vi "LabVIEW.vi"() -> ()   [LabVIEW 2022 SP3]
uses:
  <vilib>/Analysis/NI_AALBase.lvlib
  <vilib>/Analysis/baseanly.llb/Mean (DBL).vi
  Humidity_Global.vi
  <vilib>/Instr/_visa.llb/VISA Configure Serial Port (Instr).vi
panel:
  out "Fan 2":bool
  out "Gas Concentration":dbl(knob) scale=0.0..1000.0
  in  "stop 2":bool
  out "String":string
  out "Humidity":dbl
  out "Humidity Chart":dbl(graph)
  out "Humidity 2":dbl(knob) scale=0.0..100.0
  in  "VISA resource name":refnum<visa-resource-name>="COM3"
  in  "R0 (Ohms) 2":dbl
  out "Thermometer 2":dbl(slide) scale=0.0..100.0
  out "Temperature 2":dbl
  out "Temperature 3":dbl(graph)
  out "Gas Sensor Chart 3":dbl(graph)
  out "Gas Concentration 4":dbl
  out "Raw Gas Voltage":dbl
  out "Voltage In":dbl
  in  "stop":bool
  in  "Cooling ON Threshold":dbl
  in  "Cooling OFF Threshold":dbl
  out "Peltier ON":bool
  out "Fan ON":bool
  in  "Ring":u16(ring) items=["fruits", "vegetables", "fish", "meat", "dairy"]
  out "data out":string
  out "Spoiled":bool
  out "Buzzer":bool
  out "Fresh":bool
  out "Moderate":bool
  out "COOLING":string
  out "EXHAUST":string
  out "STATUS":string
  # "Smart Food Spoilage Detection System"
  # "Humidity Sensor"
  # "Temperature Sensor"
  # "Gas Sensor"
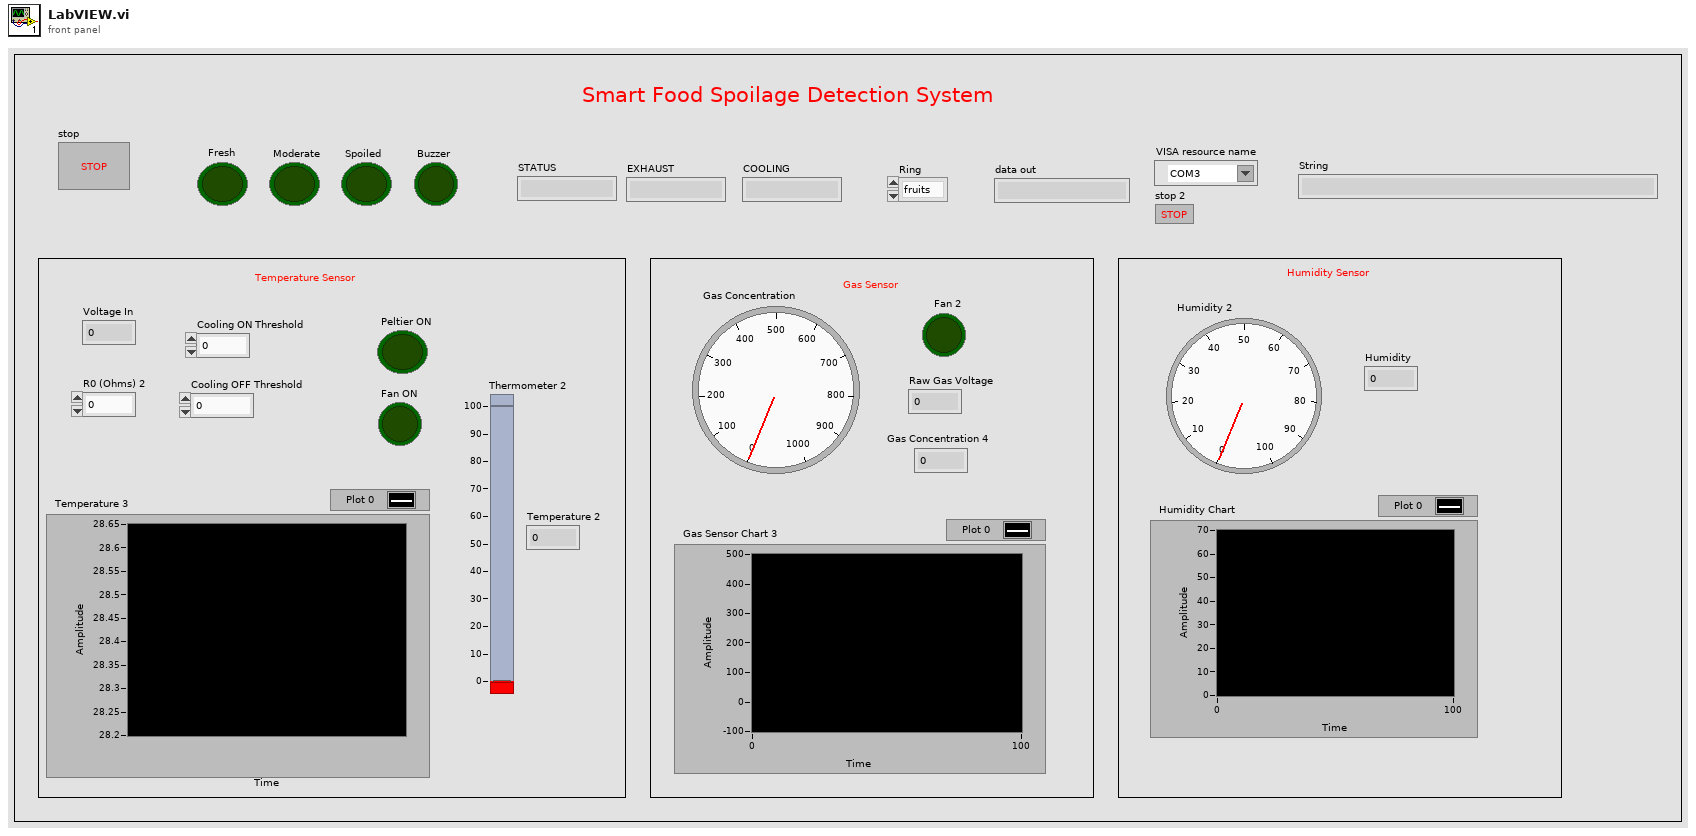
[diagram p1: front panel]
types:
  T1 = enum16{"Standard", "Buffered", "CRLF", "Immediate"}
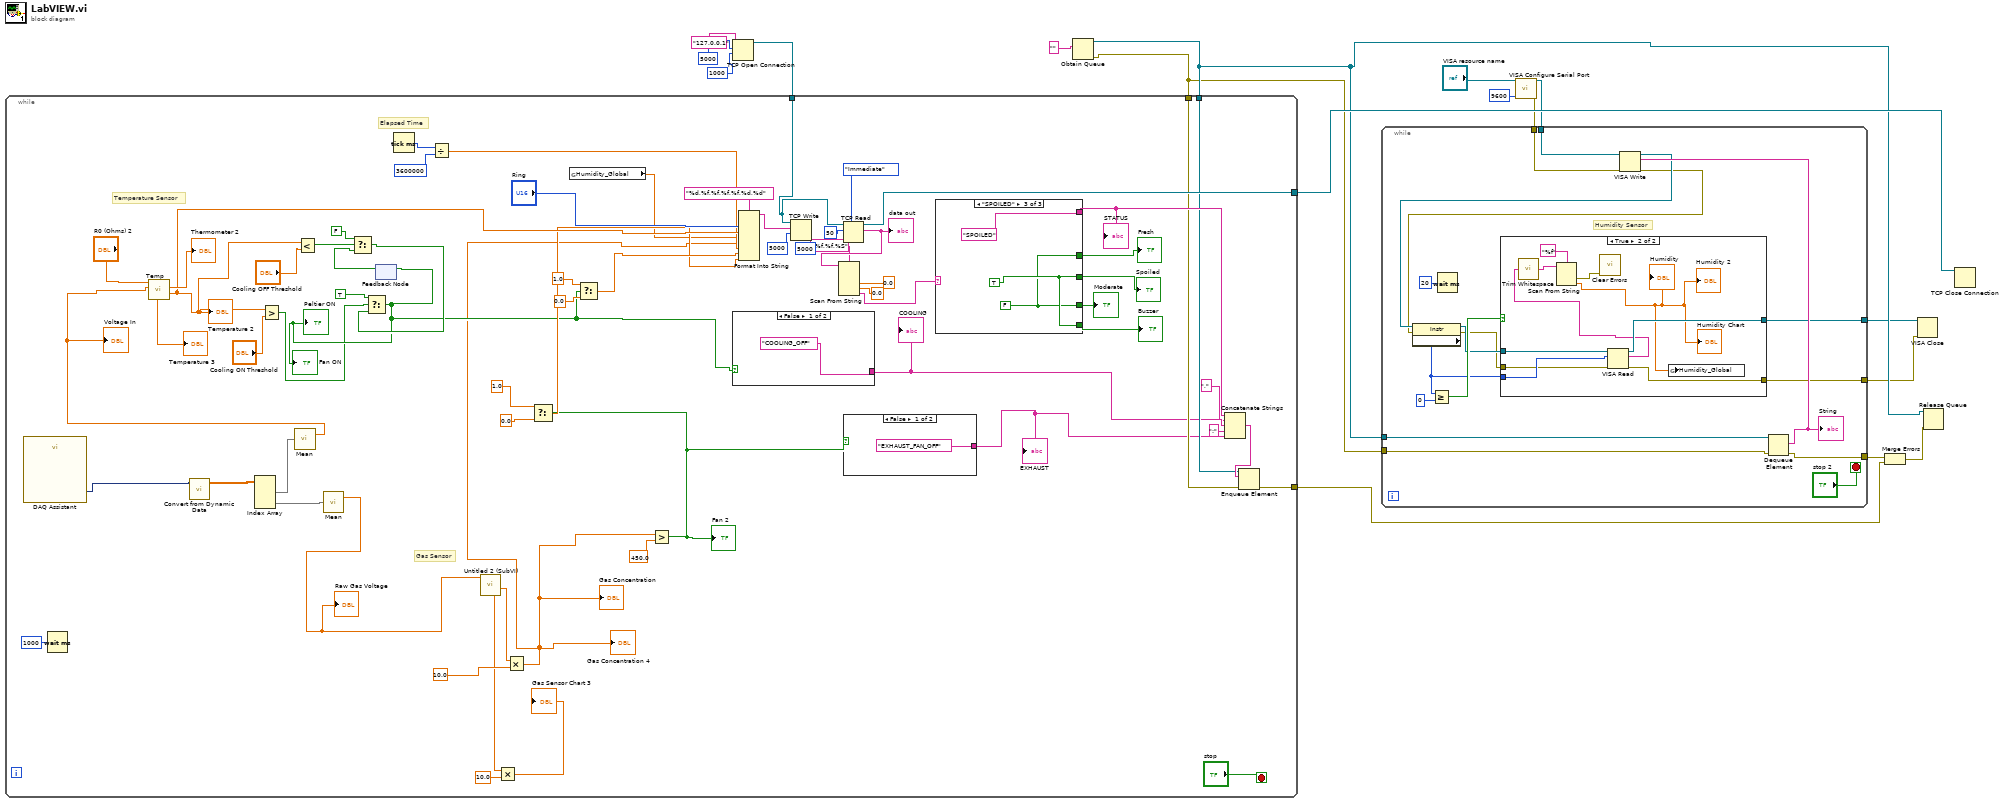
[diagram p0: block diagram]
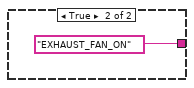
[diagram p3: hidden frame]
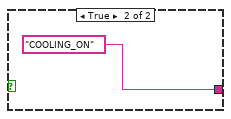
[diagram p4: hidden frame]
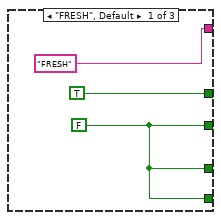
[diagram p5: hidden frame]
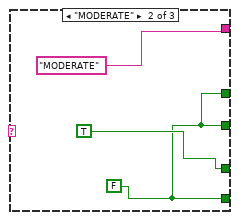
[diagram p6: hidden frame]
diagram:
  n1 = TCP Open Connection(address="127.0.0.1", remote port or service name=u16 5000, timeout ms (60000)=1000) -> (connection ID=w14:refnum<k5>)  [unwired: 2 in, 1 out]
  n2 = Obtain Queue(element data type="") -> (queue out=w9:refnum<queue>, error out=w8:errorcluster)  [unwired: 4 in, 1 out]
  n3 = while {
    tunnel: w14 -> [w35]
    tunnel: [w34] -> w12
    tunnel: w9 -> [w30]
    tunnel: w8 -> [w28]
    tunnel: [w27] -> w6
    stop <- "stop" stop-if-true
    # "Elapsed Time"
    # "Gas Sensor"
    # "Temperature Sensor"
    n4 = call "DAQ Assistant"() -> ("data"=w60:dynamicdata)  [unwired: 16 in, 3 out]
    n5 = Wait (ms)(milliseconds to wait=u32 1000) -> ()  [unwired: 1 out]
    n6 = call "Convert from Dynamic Data"("Dynamic Data Type"=w60) -> ("Array"=w80:dbl[][])  [unwired: 3 in]
    n7 = Index Array(array=w80) -> (element #1=w64:dbl[], element #2=w65:dbl[])  [unwired: 4 in]
    n8 = call-poly <vilib>:"Mean.vi"("X"=w64) -> ("mean"=w63:dbl)  [unwired: 1 out]
    "Voltage In" <- w63
    n9 = call "Temp.vi"("Voltage Input"=w63, "R0 (Ohms)"="R0 (Ohms) 2") -> ("Temperature"=w39:dbl, "Thermometer"=→"Thermometer 2":dbl, "Temperature 2"=→"Temperature 3":dbl)  [unwired: 7 in]
    "Temperature 2" <- w39
    n10 = Greater?(x=w39, y="Cooling ON Threshold") -> (0:w18:bool)
    n11 = Less?(x=w39, y="Cooling OFF Threshold") -> (x < y?=w67:bool)
    n12 = call-poly <vilib>:"Mean.vi"("X"=w65) -> ("mean"=w19:dbl)  [unwired: 1 out]
    "Raw Gas Voltage" <- w19
    n13 = feedback #1() -> (w68:bool)  [unwired: 1 in]
    n14 = Select(t=FALSE, s=w67, f=w68) -> (s? t:f=w66:bool)
    n15 = Select(t=TRUE, s=w18, f=w66) -> (s? t:f=w36:bool)
    "Peltier ON" <- w36
    "Fan ON" <- w36
    n16 = feedback-in #1(w36) -> ()
    n17 = Tick Count (ms)() -> (millisecond timer value=w62:u32)
    n18 = Divide(x=w62, y=u32 3600000) -> (x/y=w33:dbl)
    n19 = call "Untitled 2 (SubVI).vi"("Gas Voltage In"=w19) -> ("Gas Concentration 2"=w79:dbl, "Gas Sensor Chart 2"=w77:dbl)  [unwired: 9 in]
    n20 = Multiply(x=w77, y=10.0) -> (x*y=→"Gas Sensor Chart 3":dbl)
    n21 = Multiply(x=w79, y=10.0) -> (x*y=w20:dbl)
    "Gas Concentration 4" <- w20
    "Gas Concentration" <- w20
    n22 = global read "Humidity_Global.vi" "Humidity_Global"() -> (w29:dbl)
    n23 = Select(t=1.0, s=w36, f=0.0) -> (s? t:f=w38:dbl)
    n24 = Greater?(x=w20, y=450.0) -> (0:w21:bool)
    "Fan 2" <- w21
    n25 = Select(t=1.0, s=w21, f=0.0) -> (s? t:f=w37:dbl)
    n26 = case shown="False" w36 {
      tunnel: ["COOLING_OFF" "COOLING_ON"] -> w26
      frame False {
      }
      frame True {
      }
    }
    "COOLING" <- w26
    n27 = Format Into String(format string="%d,%f,%f,%f,%f,%d,%d", "Ring", w39, w29, w20, w33, w38, w37) -> (resulting string=w55:string)  [unwired: 2 in, 1 out]
    n28 = TCP Write(connection ID=w35, data in=w55, 9:5000 ("timeout ms (25000)")) -> ()  [unwired: 1 in, 3 out]
    n29 = TCP Read(connection ID=w35, bytes to read=50, 7:T1."Immediate" ("mode (standard)"), 9:5000 ("timeout ms (25000)")) -> (connection ID out=w34:refnum<k5>, data out=w53:string)  [unwired: 1 in, 1 out]
    "data out" <- w53
    n30 = Scan From String(format string="%f,%f,%S", input string=w53, default 1=0.0 ("output 1"), default 2=0.0 ("output 2")) -> (output 3=w45:string)  [unwired: 5 in, 3 out]
    n31 = case shown="False" w21 {
      tunnel: ["EXHAUST_FAN_OFF" "EXHAUST_FAN_ON"] -> w25
      frame False {
      }
      frame True {
      }
    }
    "EXHAUST" <- w25
    n32 = case shown="\"SPOILED\"" w45 {
      tunnel: ["FRESH" "MODERATE" ("String") "SPOILED" ("String")] -> w32
      tunnel: [TRUE w91 w94] -> w44
      tunnel: [w88 w91 w95] -> w43
      tunnel: [w88 w91 w95] -> w42
      tunnel: [w88 TRUE w94] -> w41
      frame "FRESH", Default {
        w88 = FALSE
      }
      frame "MODERATE" {
        w91 = FALSE
      }
      frame "SPOILED" {
        w94 = FALSE
        w95 = TRUE
      }
    }
    "Spoiled" <- w43
    "Buzzer" <- w42
    "Fresh" <- w44
    "Moderate" <- w41
    "STATUS" <- w32
    n33 = Concatenate Strings(w32, "," ("string"), w26, ":" ("string"), w25) -> (w31:string)
    n34 = Enqueue Element(queue=w30, element=w31, error in (no error)=w28) -> (error out=w27:errorcluster)  [unwired: 1 in, 2 out]
  }
  n35 = call-poly "VISA Configure Serial Port"("VISA resource name"="VISA resource name", "baud rate (9600)"=u32 9600) -> ("VISA resource name out"=w4:refnum<visa-resource-name>, "error out"=w3:errorcluster)  [unwired: 12 in]
  n36 = while {
    tunnel: w9 -> [w111]
    tunnel: w8 -> [w106]
    tunnel: [w105] -> w7
    tunnel: w4 -> [w104]
    tunnel: w3 -> [w103]
    tunnel: [w98] -> w2
    tunnel: [w97] -> w1
    stop <- "stop 2" stop-if-true
    # "Humidity Sensor"
    n37 = Wait (ms)(milliseconds to wait=u32 20) -> ()  [unwired: 1 out]
    n38 = Dequeue Element(queue=w111, error in (no error)=w106) -> (element=w110:string, error out=w105:errorcluster)  [unwired: 1 in, 2 out]
    "String" <- w110
    n39 = VISA Write(VISA resource name=w104, write buffer=w110, error in (no error)=w103) -> (VISA resource name out=w102:refnum<visa-resource-name>, error out=w101:errorcluster)  [unwired: 1 out]
    n40 = property class="Instr"(reference=w102, error in=w101) -> (reference out=w100:refnum<visa-resource-name>, error out=w99:errorcluster, "Serial Settings:Number of Bytes at Serial Port"=w107:u32)
    n41 = Greater Or Equal?(x=w107, y=u32 0) -> (x >= y?=w112:bool)
    n42 = case shown="True" w112 {
      tunnel: w107 -> [_ w125]
      tunnel: w100 -> [w115 w124]
      tunnel: w99 -> [w114 w123]
      tunnel: [w115 w122] -> w98
      tunnel: [w114 w121] -> w97
      frame False {
      }
      frame True {
        n43 = VISA Read(VISA resource name=w124, byte count=w125, error in (no error)=w123) -> (VISA resource name out=w122:refnum<visa-resource-name>, read buffer=w117:string, error out=w121:errorcluster)  [unwired: 1 out]
        n44 = call <vilib>:"Trim Whitespace.vi"("string"=w117) -> ("trimmed string"=w116:string)  [unwired: 1 in]
        n45 = Scan From String(format string="%f", input string=w116) -> (error out=w118:errorcluster, output 1=w120:dbl)  [unwired: 3 in, 2 out]
        "Humidity" <- w120
        "Humidity Chart" <- w120
        "Humidity 2" <- w120
        n46 = call <vilib>:"Clear Errors.vi"("error in (no error)"=w118) -> ()  [unwired: 5 in, 2 out]
        n47 = global write "Humidity_Global.vi" "Humidity_Global"(w120) -> ()
      }
    }
  }
  n48 = Merge Errors(w7, w6) -> (w5:errorcluster)
  n49 = VISA Close(VISA resource name=w2, error in (no error)=w1) -> ()  [unwired: 1 out]
  n50 = Release Queue(queue=w9, error in (no error)=w5) -> ()  [unwired: 1 in, 3 out]
  n51 = TCP Close Connection(connection ID=w12) -> ()  [unwired: 2 in, 2 out]
